vi "Instrucciones en cmd.vi"() -> ()   [LabVIEW 2019]
panel:
  in  "stop":bool
  out "match substring":string
  out "standard output":string
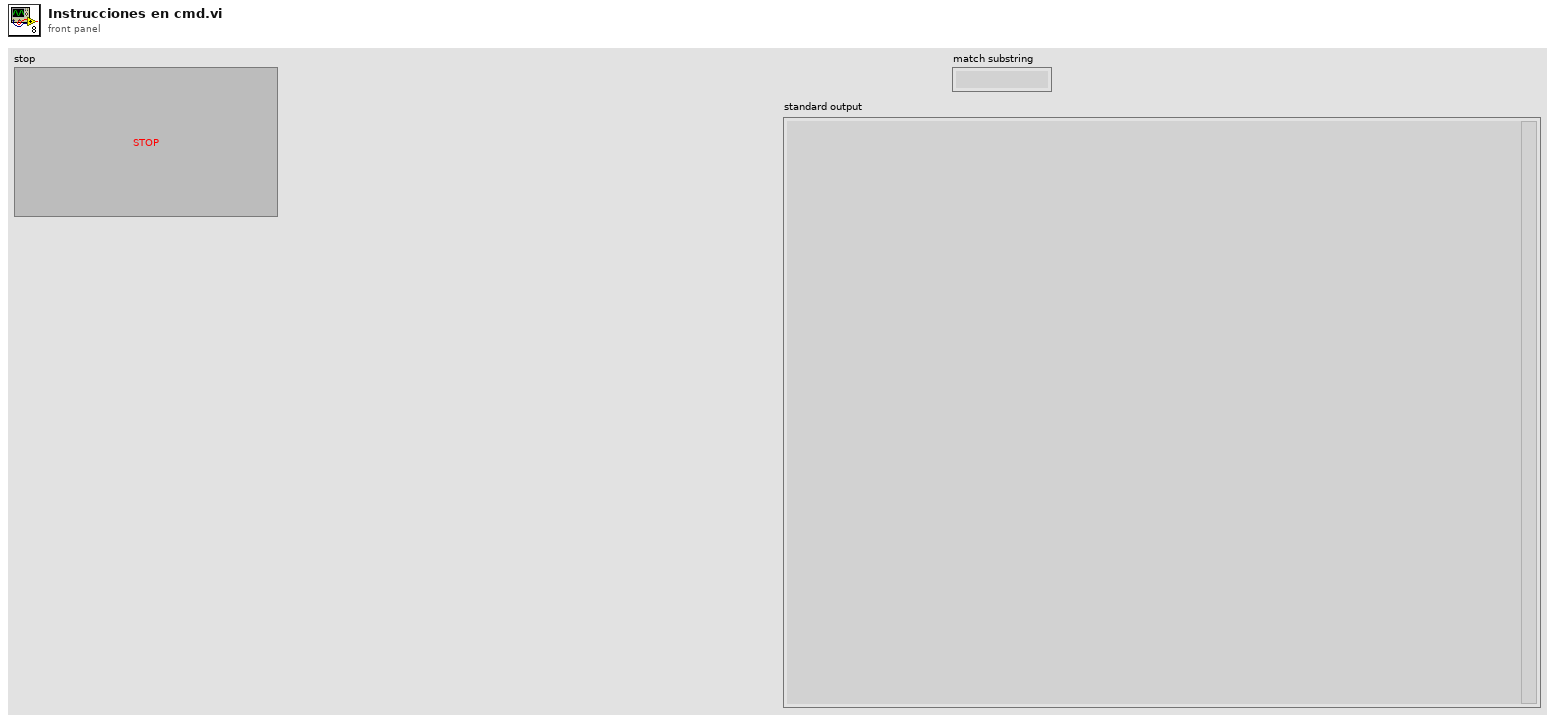
[diagram p1: front panel]
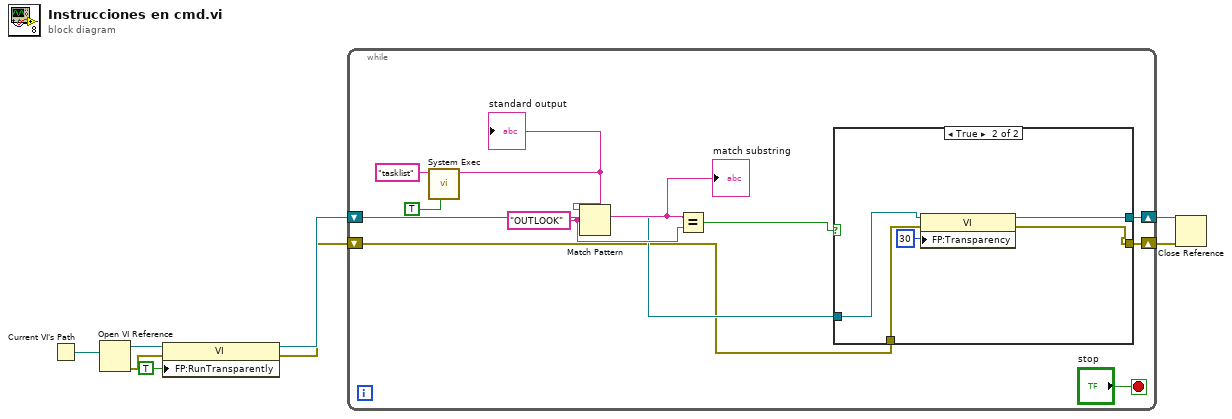
[diagram p0: block diagram]
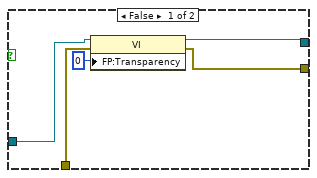
[diagram p2: hidden frame]
diagram:
  n1 = Current VI's Path() -> (path=w7:path)
  n2 = Open VI Reference(vi path=w7) -> (vi reference=w8:refnum<vi>, error out=w4:errorcluster)  [unwired: 5 in]
  n3 = property class="VI"(reference=w8, error in=w4, "FP:RunTransparently"=TRUE ("Front Panel Window:Run VI Transparently")) -> (reference out=w6:refnum<vi>, error out=w3:errorcluster)
  n4 = while {
    shift-right: [w12] -> w5
    shift-left: w6 -> [w13]
    shift-right: [w10] -> w2
    shift-left: w3 -> [w11]
    stop <- "stop" stop-if-true
    w15 = "OUTLOOK" ("regular expression")
    n5 = call <vilib>:"System Exec.vi"("run minimized? (F)"=TRUE, "command line"="tasklist") -> ("standard output"=w17:string)  [unwired: 6 in, 3 out]
    "standard output" <- w17
    n6 = Match Pattern(string=w17, regular expression=w15) -> (match substring=w16:string)  [unwired: 1 in, 3 out]
    "match substring" <- w16
    n7 = Equal?(x=w16, y=w15) -> (x = y?=w14:bool)
    n8 = case shown="True" w14 {
      tunnel: w13 -> [w23 w28]
      tunnel: [w22 w27] -> w12
      tunnel: w11 -> [w21 w26]
      tunnel: [w20 w25] -> w10
      frame False {
        n9 = property class="VI"(reference=w23, error in=w21, "FP:Transparency"=u8 0 ("Front Panel Window:Transparency")) -> (reference out=w22:refnum<vi>, error out=w20:errorcluster)
      }
      frame True {
        n10 = property class="VI"(reference=w28, error in=w26, "FP:Transparency"=u8 30 ("Front Panel Window:Transparency")) -> (reference out=w27:refnum<vi>, error out=w25:errorcluster)
      }
    }
  }
  n11 = Close Reference(reference=w5, error in (no error)=w2) -> ()  [unwired: 1 out]
